vi "反控数据上传(子VI).vi"(8 "error in (no error)":errorcluster caption="错误输入（无错误）", 11 "QN":string) -> (0 "error out":errorcluster caption="错误输出")   [LabVIEW 2016, in "数据传输系统.lvlib"]
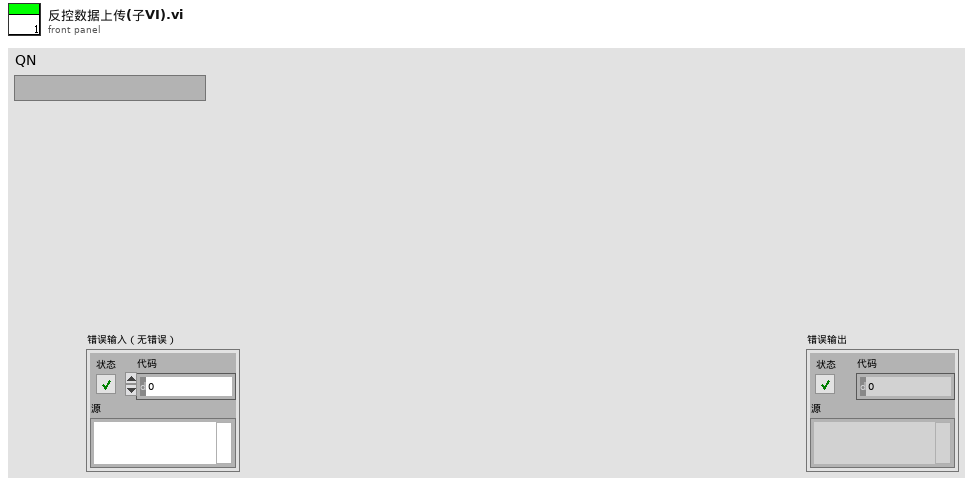
[diagram p1: front panel]
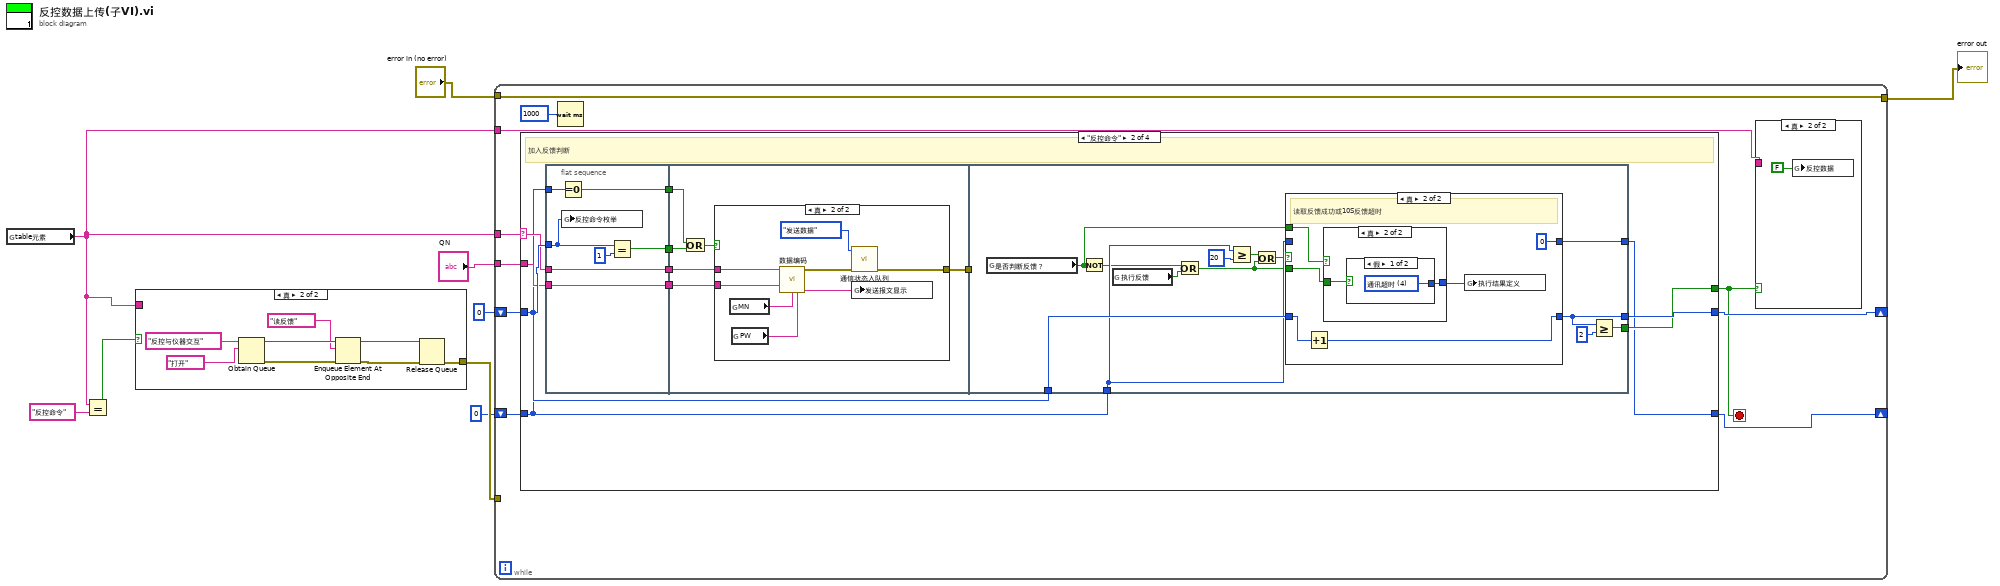
[diagram p0: block diagram]
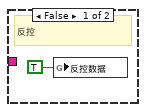
[diagram p3: hidden frame]
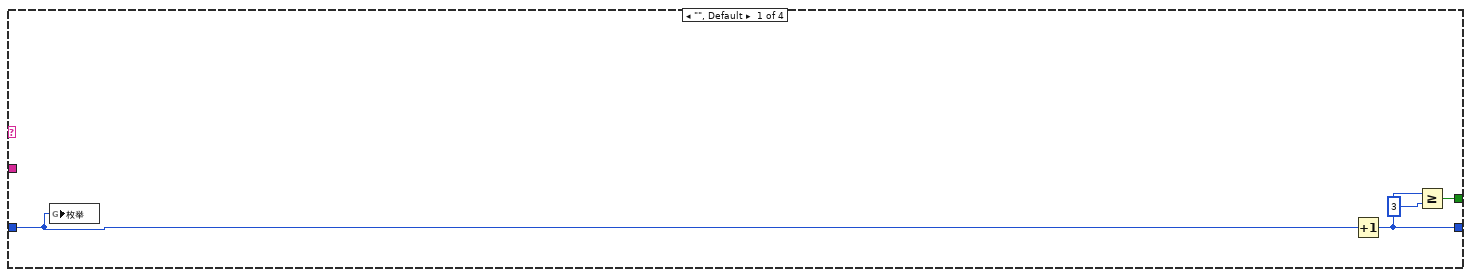
[diagram p4: hidden frame]
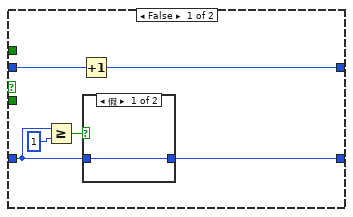
[diagram p6: hidden frame]
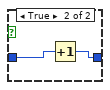
[diagram p7: hidden frame]
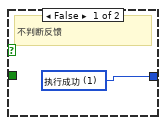
[diagram p8: hidden frame]
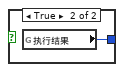
[diagram p9: hidden frame]
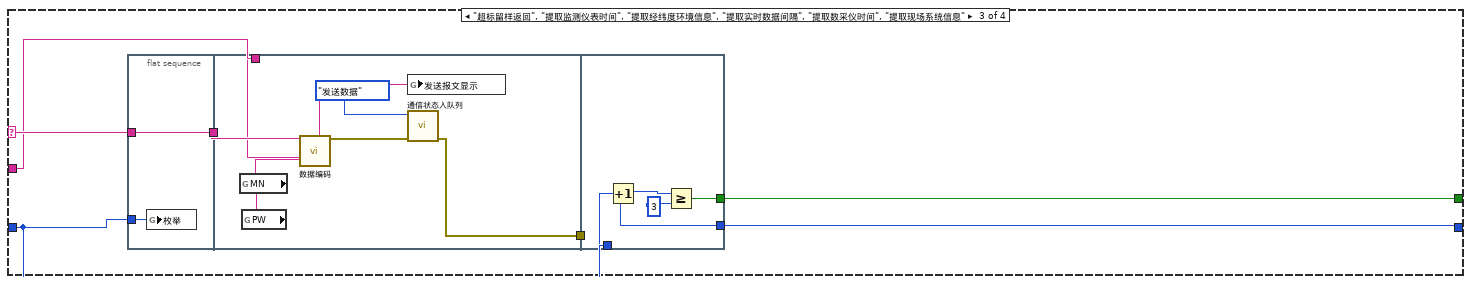
[diagram p10: hidden frame]
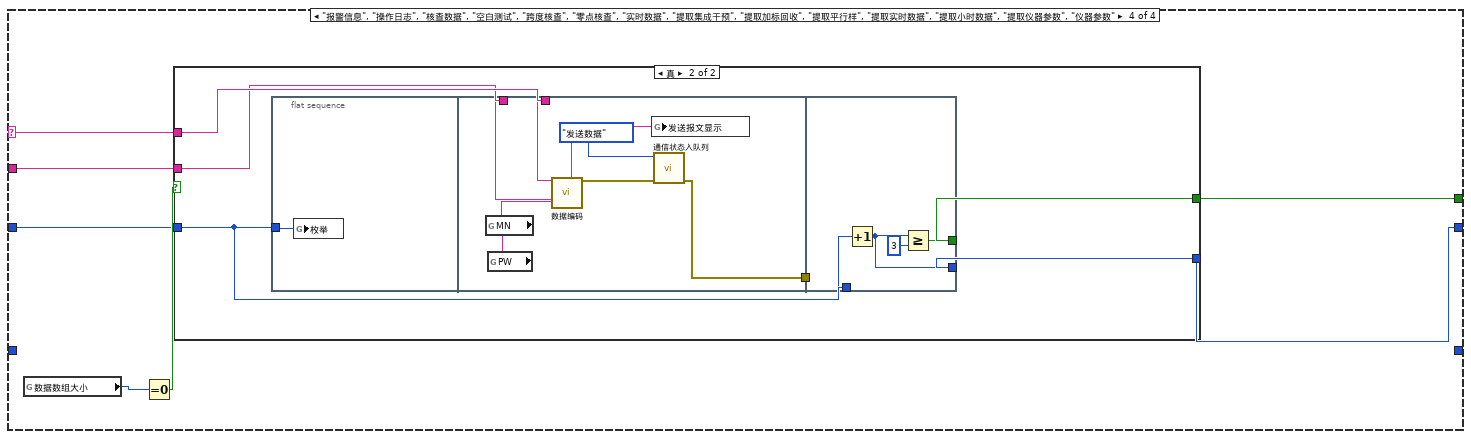
[diagram p11: hidden frame]
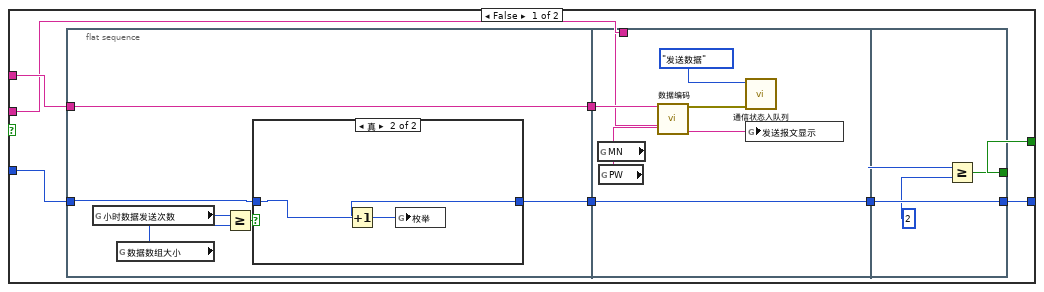
[diagram p12: hidden frame]
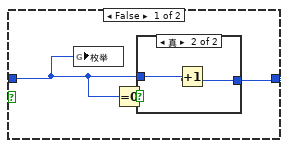
[diagram p13: hidden frame]
diagram:
  n1 = global read "全局1.vi" "table元素"() -> (w2:string)
  n2 = Equal?(x=w2, y="反控命令") -> (x = y?=w1:bool)
  n3 = case shown="真" w1 {
    tunnel: [_ w10] -> w5
    tunnel: w2 -> [_ _]
    frame False {
    }
    frame True {
      n4 = Obtain Queue(name (unnamed)="反控与仪器交互" ("名称（未命名）"), element data type="打开" ("读取写入选择")) -> (queue out=w15:refnum<queue>, error out=w14:errorcluster)  [unwired: 3 in, 1 out]
      n5 = Enqueue Element At Opposite End(queue=w15, element="读反馈" ("读取写入选择"), error in (no error)=w14) -> (queue out=w12:refnum<queue>, error out=w11:errorcluster)  [unwired: 1 in, 1 out]
      n6 = Release Queue(queue=w12, error in (no error)=w11) -> (error out=w10:errorcluster)  [unwired: 1 in, 2 out]
    }
  }
  n7 = while {
    tunnel: w2 -> [w27]
    shift-right: [w25] -> _
    shift-left: 0 -> [w26]
    tunnel: w2 -> [w23]
    tunnel: "QN" -> [w21]
    tunnel: "error in (no error)" -> [w20]
    tunnel: [w20] -> w6
    tunnel: w5 -> [_]
    shift-right: [w18] -> _
    shift-left: 0 -> [w19]
    stop <- w24 stop-if-true
    n8 = case shown="\"反控命令\"" w27 {
      selector: w27 -> [_ w42 w106 w123]
      tunnel: w26 -> [w32 w43 w103 w122]
      tunnel: [w31 w40 w102 w127] -> w24
      tunnel: [w30 w41 w101 w126] -> w25
      tunnel: w21 -> [_ w39 w100 w121]
      tunnel: w19 -> [_ w35 _ _]
      tunnel: [_ w37 _ _] -> w18
      frame "", Default {
        n9 = global write "全局1.vi" "枚举"(w32) -> ()
        n10 = Increment(x=w32) -> (x+1=w30:i32)
        n11 = Greater Or Equal?(x=w30, y=3) -> (x >= y?=w31:bool)
      }
      frame "反控命令" {
        # "加入反馈判断"
        n12 = flat-sequence {
          tunnel: w42 -> [w52]
          tunnel: [w52] -> w45
          tunnel: w43 -> [w50]
          tunnel: w39 -> [w51]
          tunnel: [w51] -> w38
          tunnel: [w48] -> w36
          tunnel: w35 -> [w47]
          tunnel: [w46] -> w34
          tunnel: w45 -> [w58]
          tunnel: [w57] -> w44
          tunnel: w38 -> [w56]
          tunnel: w36 -> [w54]
          tunnel: w34 -> [w53]
          tunnel: w44 -> [_]
          tunnel: w43 -> [w78]
          tunnel: [w77] -> w40
          tunnel: [w76] -> w41
          tunnel: w35 -> [w74]
          tunnel: [w75] -> w37
          frame #0 {
            n13 = Equal To 0?(x=w47) -> (x = 0?=w46:bool)
            n14 = global write "全局 反控命令枚举.vi" "反控命令枚举"(w50) -> ()
            n15 = Equal?(x=w50, y=1) -> (x = y?=w48:bool)
          }
          frame #1 {
            n16 = Or(x=w53, y=w54) -> (x .or. y?=w55:bool)
            n17 = case shown="真" w55 {
              tunnel: w58 -> [_ w61]
              tunnel: [_ w60] -> w57
              tunnel: w56 -> [_ w59]
              frame False {
              }
              frame True {
                n18 = global read "断电保存全局.vi" "MN"() -> (w66:string)
                n19 = global read "断电保存全局.vi" "PW"() -> (w65:string)
                n20 = call "数据编码.vi"("table输入"=w61, "QN"=w59, "MN"=w66, "PW"=w65) -> ("错误常量"=w63:errorcluster, "通讯包字符串"=w64:string)  [unwired: 10 in]
                n21 = call "通信状态入队列.vi"("错误输入（无错误）"=w63, "枚举"=enum16{"打开连接", "发送数据", "读取数据", "数据处理", "关闭连接"}."发送数据") -> ("错误输出"=w60:errorcluster)  [unwired: 9 in]
                n22 = global write "全局1.vi" "发送报文显示"(w64) -> ()
              }
            }
          }
          frame #2 {
            n23 = global read "全局 反控命令枚举.vi" "是否判断反馈？"() -> (w67:bool)
            n24 = Not(x=w67) -> (.not. x?=w68:bool)
            n25 = global read "全局 反控命令枚举.vi" "执行反馈"() -> (w70:bool)
            n26 = Or(x=w68, y=w70) -> (x .or. y?=w69:bool)
            n27 = Greater Or Equal?(x=w74, y=20) -> (x >= y?=w71:bool)
            n28 = Or(x=w71, y=w69) -> (x .or. y?=w72:bool)
            n29 = case shown="真" w72 {
              tunnel: w78 -> [w81 w94]
              tunnel: [w80 w93] -> w76
              tunnel: w74 -> [w85 _]
              tunnel: [w84 0] -> w75
              tunnel: w69 -> [_ w92]
              tunnel: w67 -> [_ w90]
              frame False {
                n30 = Greater Or Equal?(x=w81, y=1) -> (x >= y?=w82:bool)
                n31 = Increment(x=w85) -> (x+1=w84:i32)
                n32 = case shown="假" w82 {
                  tunnel: w81 -> [w86 w88]
                  tunnel: [w86 w87] -> w80
                  frame False {
                  }
                  frame True {
                    n33 = Increment(x=w88) -> (x+1=w87:i32)
                  }
                }
              }
              frame True {
                # "读取反馈成功或10S反馈超时"
                n34 = Increment(x=w94) -> (x+1=w93:i32)
                n35 = case shown="真" w90 {
                  tunnel: w92 -> [_ w97]
                  tunnel: [w95 w96] -> w89
                  frame False {
                    w95 = u16 1 items=["执行成功"=1, "执行失败，但不知道原因"=2, "命令请求条件错误"=3, "通讯超时"=4, "系统繁忙不能执行"=5, "系统故障"=6, "没有数据"=100] ("执行结果定义")
                    # "不判断反馈"
                  }
                  frame True {
                    n36 = case shown="假" w97 {
                      tunnel: [w98 w99] -> w96
                      frame False {
                        w98 = u16 4 items=["执行成功"=1, "执行失败，但不知道原因"=2, "命令请求条件错误"=3, "通讯超时"=4, "系统繁忙不能执行"=5, "系统故障"=6, "没有数据"=100] ("执行结果定义")
                      }
                      frame True {
                        n37 = global read "全局 反控命令枚举.vi" "执行结果"() -> (w99:u16)
                      }
                    }
                  }
                }
                n38 = global write "全局 反控命令枚举.vi" "执行结果定义"(w89) -> ()
              }
            }
            n39 = Greater Or Equal?(x=w76, y=2) -> (x >= y?=w77:bool)
          }
        }
      }
      frame "超标留样返回", "提取监测仪表时间", "提取经纬度环境信息", "提取实时数据间隔", "提取数采仪时间", "提取现场系统信息" {
        n40 = flat-sequence {
          tunnel: w106 -> [w108]
          tunnel: [w108] -> w105
          tunnel: w103 -> [w107]
          tunnel: w105 -> [w111]
          tunnel: [w110] -> w104
          tunnel: w100 -> [w109]
          tunnel: w104 -> [_]
          tunnel: w103 -> [w119]
          tunnel: [w118] -> w102
          tunnel: [w117] -> w101
          frame #0 {
            n41 = global write "全局1.vi" "枚举"(w107) -> ()
          }
          frame #1 {
            n42 = global read "断电保存全局.vi" "MN"() -> (w116:string)
            n43 = global read "断电保存全局.vi" "PW"() -> (w115:string)
            n44 = call "数据编码.vi"("table输入"=w111, "QN"=w109, "MN"=w116, "PW"=w115) -> ("错误常量"=w113:errorcluster, "通讯包字符串"=w114:string)  [unwired: 10 in]
            n45 = global write "全局1.vi" "发送报文显示"(w114) -> ()
            n46 = call "通信状态入队列.vi"("错误输入（无错误）"=w113, "枚举"=enum16{"打开连接", "发送数据", "读取数据", "数据处理", "关闭连接"}."发送数据") -> ("错误输出"=w110:errorcluster)  [unwired: 9 in]
          }
          frame #2 {
            n47 = Increment(x=w119) -> (x+1=w117:i32)
            n48 = Greater Or Equal?(x=w117, y=3) -> (x >= y?=w118:bool)
          }
        }
      }
      frame "报警信息", "操作日志", "核查数据", "空白测试", "跨度核查", "零点核查", "实时数据", "提取集成干预", "提取加标回收", "提取平行样", "提取实时数据", "提取小时数据", "提取仪器参数", "仪器参数" {
        n49 = global read "全局 数据数组大小.vi" "数据数组大小"() -> (w125:i32)
        n50 = Equal To 0?(x=w125) -> (x = 0?=w124:bool)
        n51 = case shown="真" w124 {
          tunnel: [w132 w162] -> w127
          tunnel: [w131 w163] -> w126
          tunnel: w123 -> [w130 w165]
          tunnel: w122 -> [w129 w164]
          tunnel: w121 -> [w128 w161]
          frame False {
            n52 = flat-sequence {
              tunnel: w129 -> [w138]
              tunnel: [w136] -> w135
              tunnel: w130 -> [w137]
              tunnel: [w137] -> w134
              tunnel: w135 -> [w157]
              tunnel: [w157] -> w133
              tunnel: w134 -> [w151]
              tunnel: w128 -> [w150]
              tunnel: w133 -> [w160]
              tunnel: [w160] -> w131
              tunnel: [w159] -> w132
              frame #0 {
                n53 = global read "全局 小时数据发送次数.vi" "小时数据发送次数"() -> (w140:i32)
                n54 = global read "全局 数据数组大小.vi" "数据数组大小"() -> (w141:i32)
                n55 = Greater Or Equal?(x=w140, y=w141) -> (x >= y?=w139:bool)
                n56 = case shown="真" w139 {
                  tunnel: w138 -> [w143 w149]
                  tunnel: [w144 w148] -> w136
                  frame False {
                    n57 = global write "全局1.vi" "枚举"(w143) -> ()
                    n58 = Equal To 0?(x=w143) -> (x = 0?=w142:bool)
                    n59 = case shown="真" w142 {
                      tunnel: w143 -> [w145 w147]
                      tunnel: [w145 w146] -> w144
                      frame False {
                      }
                      frame True {
                        n60 = Increment(x=w147) -> (x+1=w146:i32)
                      }
                    }
                  }
                  frame True {
                    n61 = Increment(x=w149) -> (x+1=w148:i32)
                    n62 = global write "全局1.vi" "枚举"(w148) -> ()
                  }
                }
              }
              frame #1 {
                n63 = global read "断电保存全局.vi" "MN"() -> (w152:string)
                n64 = global read "断电保存全局.vi" "PW"() -> (w153:string)
                n65 = call "数据编码.vi"("table输入"=w151, "QN"=w150, "MN"=w152, "PW"=w153) -> ("错误常量"=w155:errorcluster, "通讯包字符串"=w154:string)  [unwired: 10 in]
                n66 = call "通信状态入队列.vi"("错误输入（无错误）"=w155, "枚举"=enum16{"打开连接", "发送数据", "读取数据", "数据处理", "关闭连接"}."发送数据") -> ()  [unwired: 9 in, 1 out]
                n67 = global write "全局1.vi" "发送报文显示"(w154) -> ()
              }
              frame #2 {
                n68 = Greater Or Equal?(x=w160, y=2) -> (x >= y?=w159:bool)
              }
            }
          }
          frame True {
            n69 = flat-sequence {
              tunnel: w164 -> [w167]
              tunnel: [w170] -> w166
              tunnel: w165 -> [w169]
              tunnel: w161 -> [w168]
              tunnel: w166 -> [_]
              tunnel: [w178] -> w162
              tunnel: [w177] -> w163
              tunnel: w164 -> [w176]
              frame #0 {
                n70 = global write "全局1.vi" "枚举"(w167) -> ()
              }
              frame #1 {
                n71 = global read "断电保存全局.vi" "MN"() -> (w175:string)
                n72 = global read "断电保存全局.vi" "PW"() -> (w174:string)
                n73 = call "数据编码.vi"("table输入"=w169, "QN"=w168, "MN"=w175, "PW"=w174) -> ("错误常量"=w172:errorcluster, "通讯包字符串"=w173:string)  [unwired: 10 in]
                n74 = global write "全局1.vi" "发送报文显示"(w173) -> ()
                n75 = call "通信状态入队列.vi"("错误输入（无错误）"=w172, "枚举"=enum16{"打开连接", "发送数据", "读取数据", "数据处理", "关闭连接"}."发送数据") -> ("错误输出"=w170:errorcluster)  [unwired: 9 in]
              }
              frame #2 {
                n76 = Increment(x=w176) -> (x+1=w177:i32)
                n77 = Greater Or Equal?(x=w177, y=3) -> (x >= y?=w178:bool)
              }
            }
          }
        }
      }
    }
    n78 = Wait (ms)(milliseconds to wait=u32 1000 ("等待时间（毫秒）")) -> ()  [unwired: 1 out]
    n79 = case shown="真" w24 {
      tunnel: w23 -> [_ _]
      frame False {
        # "反控"
        n80 = global write "全局1.vi" "反控数据"(TRUE ("反控数据")) -> ()
      }
      frame True {
        n81 = global write "全局1.vi" "反控数据"(FALSE ("反控数据")) -> ()
      }
    }
  }
  "error out" <- w6
